vi "TypeDescriptor_ExtractDescriptorElements.vi"(9 "Data String":string, 11 "type descriptor":i16[](array[numeric]) format="%04x") -> (0 "concatenated element descriptors":i16[](array[numeric]), 1 "Nb elements":i32, 2 "elements":T1[](array[typedef]), 3 "type descriptor dup":i16[](array[numeric]) format="%.0x")   [LabVIEW 2020, in "OpenDescriptor.lvlib"]
uses:
  OpenDescriptor.lvlib
  OpenDescriptor -- cluster.ctl
  TypeDescriptor_GetPString.vi
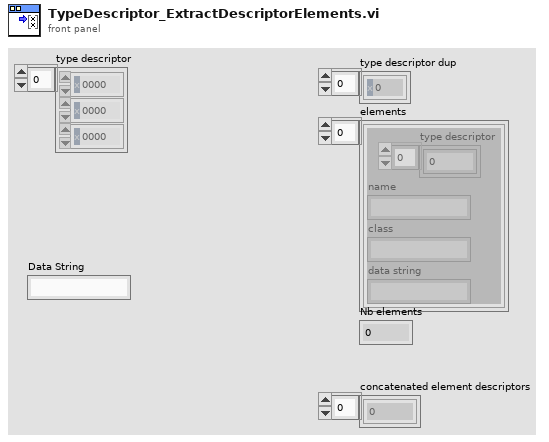
[diagram p1: front panel]
types:
  T1 = typedef "OpenDescriptor.lvlib/OpenDescriptor -- cluster.ctl" = cluster{"type descriptor":i16[], "name":string, "class":string, "data string":string}
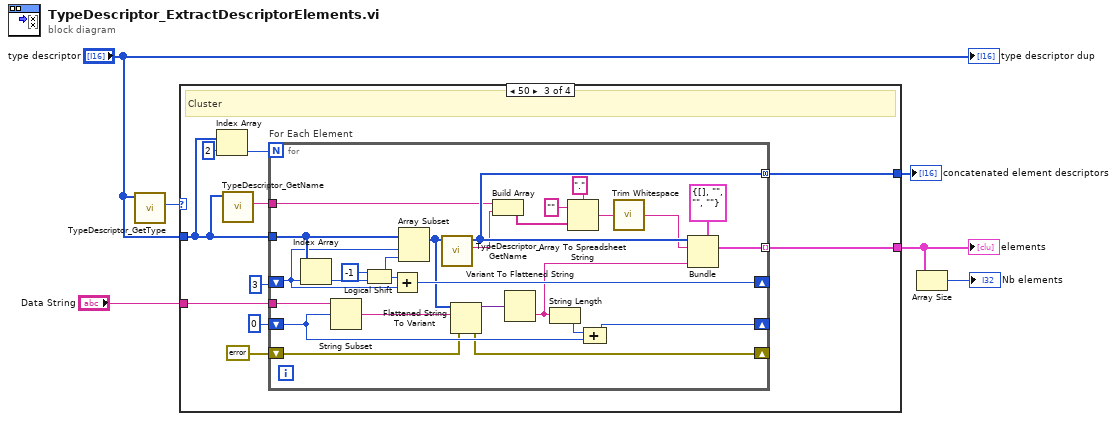
[diagram p0: block diagram]
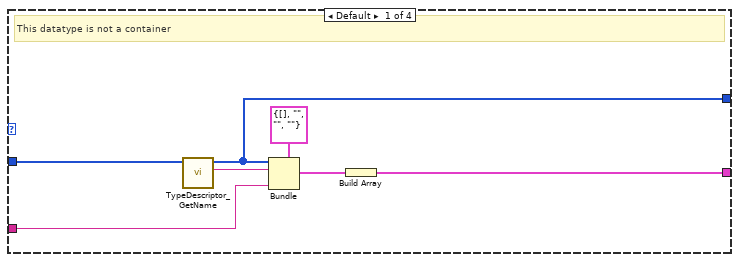
[diagram p2: hidden frame]
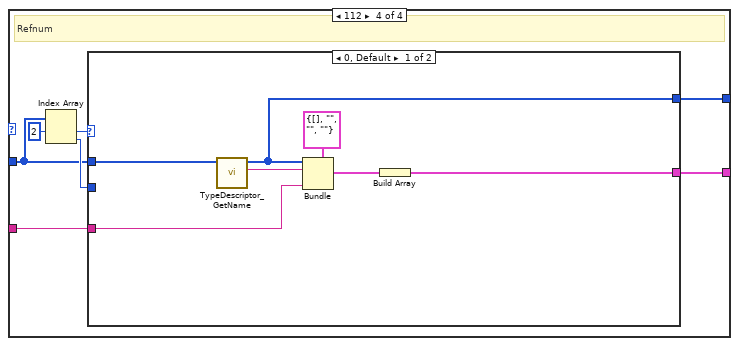
[diagram p4: hidden frame]
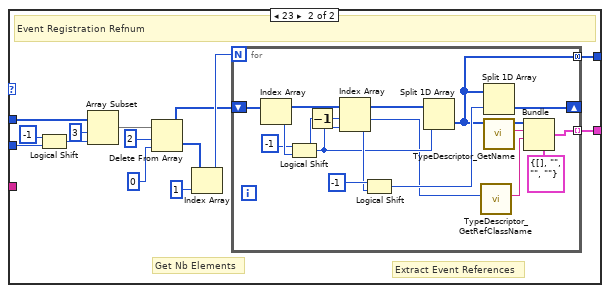
[diagram p5: hidden frame]
diagram:
  n1 = call "TypeDescriptor_GetType.vi"("type descriptor"="type descriptor") -> ("Type"=w5:u8)  [unwired: 9 in, 1 out]
  n2 = case shown="50" w5 {
    tunnel: [w9 _ w20 w52] -> w4
    tunnel: "type descriptor" -> [w11 _ w15 w53]
    tunnel: [w8 _ w19 w51] -> w2
    tunnel: "Data String" -> [w7 _ w17 w50]
    frame Default {
      # "This datatype is not a container"
      n3 = call "TypeDescriptor_GetName.vi"("type descriptor"=w11) -> ("name"=w13:string, "type descriptor dup"=w8:i16[])  [unwired: 8 in, 1 out]
      n4 = Bundle(cluster=T1 {"type descriptor"=[], "name"="", "class"="", "data string"=""} ("Descriptor Element"), "type descriptor"=w8, "name"=w13, "data string"=w7) -> (w10:T1)  [unwired: 1 in]
      n5 = Build Array(w10) -> (w9:T1[])
    }
    frame 0 {
      # "void"
    }
    frame 80 {
      # "Cluster"
      n6 = Index Array(array=w15, index=2) -> (element=w22:i16)
      n7 = call "TypeDescriptor_GetName.vi"("type descriptor"=w15) -> ("name"=w14:string)  [unwired: 8 in, 2 out]
      n8 = for "For Each Element" {
        N: w22 -> [_]
        tunnel: w15 -> [w46]
        shift-right: [w47] -> _
        shift-left: 3 ("index") -> [w45]
        tunnel: [w43] -> w20 mode=indexing
        tunnel: [w41] -> w19 mode=concatenating
        shift-right: [w34] -> _
        shift-left: 0 -> [w35]
        tunnel: w17 -> [w40]
        shift-right: [w31] -> _
        shift-left: errorcluster {"status"=FALSE, "code"=0, "source"=""} ("error out") -> [w32]
        tunnel: w14 -> [w30]
        n9 = Index Array(array=w46, index=w45) -> (element=w48:i16)
        n10 = String Subset(string=w40, offset (0)=w35) -> (substring=w38:string)  [unwired: 1 in]
        n11 = Logical Shift(y=i16 -1, x=w48) -> (x << y=w44:i16)
        n12 = Add(x=w44, y=w45) -> (x+y=w47:i32)
        n13 = Array Subset(array=w46, index=w45, length=w44) -> (w39:i16[])
        n14 = call "TypeDescriptor_GetName.vi"("type descriptor"=w39) -> ("name"=w29:string, "type descriptor dup"=w41:i16[])  [unwired: 8 in, 1 out]
        n15 = Flattened String To Variant(4:w32, 6:w38, 7:w39) -> (0:w31:errorcluster, 3:w37:variant)
        n16 = Build Array(w30, w29) -> (w25:string[])
        n17 = Variant To Flattened String(Variant=w37) -> (data string=w33:string)  [unwired: 1 out]
        n18 = String Length(string=w33) -> (length=w36:i32)
        n19 = Array To Spreadsheet String(delimiter (Tab)=".", array=w25, 3:"" ("format string")) -> (spreadsheet string=w28:string)
        n20 = Compound Arithmetic op=ADD(w36, w35) -> (w34:i32)
        n21 = call <vilib>:"Trim Whitespace.vi"("string"=w28) -> ("trimmed string"=w24:string)  [unwired: 1 in]
        n22 = Bundle(cluster=T1 {"type descriptor"=[], "name"="", "class"="", "data string"=""} ("Descriptor Element"), "type descriptor"=w41, "name"=w24, "data string"=w33) -> (w43:T1)  [unwired: 1 in]
      }
    }
    frame 112 {
      # "Refnum"
      n23 = Index Array(array=w53, index #1=2 ("index")) -> (element #1=w55:i16, element #2=w54:i16)  [unwired: 1 in]
      n24 = case shown="0, Default" w55 {
        tunnel: w54 -> [_ w74]
        tunnel: w53 -> [w60 w77]
        tunnel: [w58 w65] -> w52
        tunnel: [w59 w64] -> w51
        tunnel: w50 -> [w57 _]
        frame 0, Default {
          n25 = call "TypeDescriptor_GetName.vi"("type descriptor"=w60) -> ("name"=w61:string, "type descriptor dup"=w59:i16[])  [unwired: 8 in, 1 out]
          n26 = Bundle(cluster=T1 {"type descriptor"=[], "name"="", "class"="", "data string"=""} ("Descriptor Element"), "type descriptor"=w59, "name"=w61, "data string"=w57) -> (w63:T1)  [unwired: 1 in]
          n27 = Build Array(w63) -> (w58:T1[])
        }
        frame 23 {
          # "Extract Event References"
          # "Get Nb Elements"
          # "Event Registration Refnum"
          n28 = Logical Shift(y=i16 -1, x=w74) -> (x << y=w73:i16)
          n29 = Array Subset(array=w77, index=3, length=w73) -> (w72:i16[])
          n30 = Delete From Array(array=w72, length=2 ("index"), index=0) -> (deleted portion=w70:i16[], array with subset deleted=w66:i16[])
          n31 = Index Array(array=w70, index=1) -> (element=w67:i16)
          n32 = for {
            N: w67 -> [_]
            shift-right: [w85] -> _
            shift-left: w66 -> [w88]
            tunnel: [w80] -> w65 mode=indexing
            tunnel: [w78] -> w64 mode=concatenating
            n33 = Index Array(array=w88) -> (element=w93:i16)  [unwired: 1 in]
            n34 = Logical Shift(y=i16 -1, x=w93) -> (x << y=w87:i16)
            n35 = Decrement(x=w87) -> (x-1=w89:i16)
            n36 = Index Array(array=w88, index #1=w89, index #2=w87) -> (element #1=w84:i16, element #2=w90:i16)
            n37 = Logical Shift(y=i16 -1, x=w90) -> (x << y=w86:i16)
            n38 = Split 1D Array(array=w88, index=w87) -> (second subarray=w78:i16[])  [unwired: 1 out]
            n39 = call "TypeDescriptor_GetRefClassName.vi"("Ref Class"=w84) -> ("Reference Class"=w82:string)  [unwired: 10 in]
            n40 = Split 1D Array(array=w78, index=w86) -> (second subarray=w85:i16[])  [unwired: 1 out]
            n41 = call "TypeDescriptor_GetName.vi"("type descriptor"=w78) -> ("name"=w81:string, "type descriptor dup"=w83:i16[])  [unwired: 8 in, 1 out]
            n42 = Bundle(cluster=T1 {"type descriptor"=[], "name"="", "class"="", "data string"=""} ("Descriptor Element"), "type descriptor"=w83, "name"=w81, "class"=w82) -> (w80:T1)  [unwired: 1 in]
          }
        }
      }
    }
  }
  "elements" <- w4
  "concatenated element descriptors" <- w2
  n43 = Array Size(array=w4) -> (size(s)=→"Nb elements":i32)
  "type descriptor dup" <- "type descriptor"
